vi "validate.vi"(8 "error in":errorcluster, 11 "configuration in":refnum<class "fixed channel configuration.lvclass">) -> (0 "error out":errorcluster, 3 "configuration out":refnum<class "fixed channel configuration.lvclass">)   [LabVIEW 2013, in "fixed channel configuration.lvclass"]
doc: "Provides an interface for performing validation on a given configuration. Any children should define the behavior of this function to ensure that the configuration in memory can be used by the runtime class."
uses:
  fixed channel configuration.lvclass
  <vilib>/NI/Tag Bus Module Framework/module configuration/TBM module configuration.lvclass
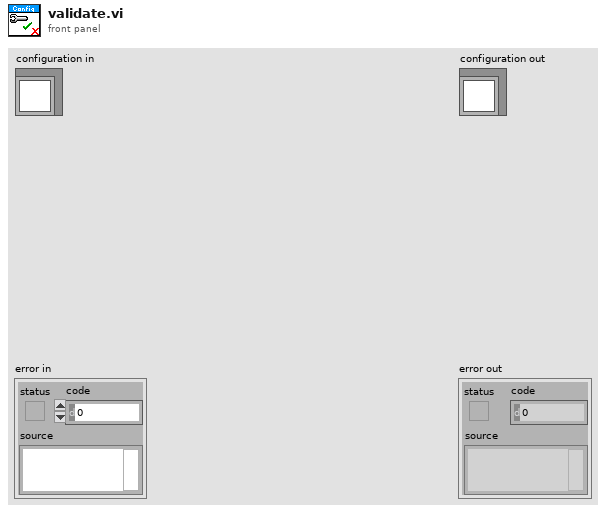
[diagram p1: front panel]
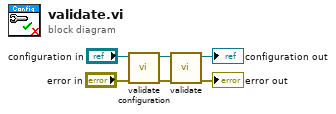
[diagram p0: block diagram]
diagram:
  n1 = call-dynamic "validate configuration.vi"("error in"="error in", "fixed channel configuration in"="configuration in") -> ("error out"=w3:errorcluster, "fixed channel configuration out"=w1:refnum<class "fixed channel configuration.lvclass">)  [unwired: 8 in]
  n2 = call-parent "validate.vi"("error in"=w3, "configuration in"=w1) -> ("error out"=→"error out":errorcluster, "configuration out"=→"configuration out":refnum<class "fixed channel configuration.lvclass">)  [unwired: 8 in]
